vi "zStack.vi"() -> ()   [LabVIEW 2015]
panel:
  in  "642 nm filter":T1(ring)=enum."665/LP [Cy5]"
  in  "561 nm filter":T1(ring)=enum."605/70 [Cy3]"
  in  "488 nm filter":T1(ring)=enum."525/50 [FITC]"
  in  "405 nm filter":T1(ring)
  in  "Filter wheel init":cluster{"FW Handle":u32, "init?":i16}
  in  "Z stage":T2
  in  "XY stage":T3
  in  "sCMOS init":cluster{"init":i16, "sCMOS handle":u32}
  in  "405 nm (aq)":bool=TRUE
  in  "488 nm (aq)":bool=TRUE
  in  "561 nm (aq)":bool=TRUE
  in  "642 nm (aq)":bool=TRUE
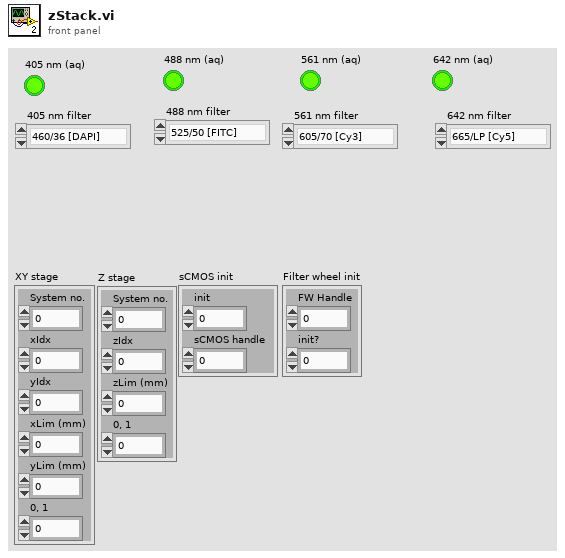
[diagram p1: front panel]
types:
  T1 = enum16{"460/36 [DAPI]", "525/50 [FITC]", "605/70 [Cy3]", "665/LP [Cy5]", "Empty-1", "Empty-2"}
  T2 = cluster{"System no.":i32, "zIdx":i32, "zLim (mm)":dbl, "0, 1":i16}
  T3 = cluster{"System no.":i32, "xIdx":i32, "yIdx":i32, "xLim (mm)":dbl, "yLim (mm)":dbl, "0, 1":i16}
  T4 = cluster{"Component ID":string, "COM Port":refnum<visa-resource-name>, "Type ":enum16{"omicronLuxX", "coherentObis"}, "init":i16}[]
  T5 = enum16{"460/36 [DAPI]", "525/50 [FITC]", "605/70 [Cy3]", "665/LP [Cy5]", "Empty-1", "Empty-2"}[]
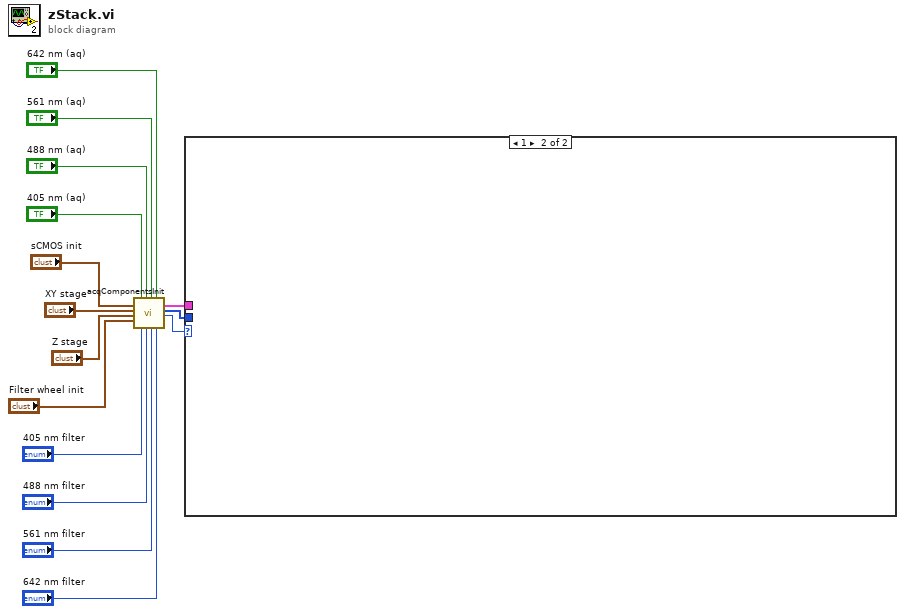
[diagram p0: block diagram]
diagram:
  n1 = call "acqComponentsInit.vi"("sCMOS init"="sCMOS init", "XY stage"="XY stage", "Z stage"="Z stage", "Filter wheel init"="Filter wheel init", "405 nm (aq)"="405 nm (aq)", "405 nm filter"="405 nm filter", "488 nm (aq)"="488 nm (aq)", "488 nm filter"="488 nm filter", "561 nm (aq)"="561 nm (aq)", "561 nm filter"="561 nm filter", "642 nm (aq)"="642 nm (aq)", "642 nm filter"="642 nm filter") -> ("initializedLasers"=w2:T4, "Initialized filters"=w1:T5, "correctCompInit?"=w3:i32)  [unwired: 5 in]
  n2 = case shown="1" w3 {
    tunnel: w2 -> [_ _]
    tunnel: w1 -> [_ _]
    frame 0, Default {
    }
    frame 1 {
    }
  }
